vi "Write Clone name.vi"(8 "error in (no error)":errorcluster, 10 "Clone name":string, 11 "Fiber Auto Collimation panel in":refnum<class "Fiber Auto Collimation panel.lvclass">) -> (0 "error out":errorcluster, 3 "Fiber Auto Collimation panel out":refnum<class "Fiber Auto Collimation panel.lvclass">)   [LabVIEW 2018, in "Fiber Auto Collimation panel.lvclass"]
doc: "The \"Clone name\" is only needed if this is a Panel class that can be open more than once. If the panel will only be open once at a time, don't bother using this element of the private data for anything.\n\nClone names are forced into lower case and have whitespace removed from them when written. If the panel can be open more than once simultaneously, just be sure that each instance of the panel has a unique non-blank name.\n\nNote: The clone name should only be written during the panel launch and then propagated appropriately afterwards. Do not change the clone name after the panel has been started!"
uses:
  Fiber Auto Collimation panel.lvclass
  Fiber Auto Collimation panel.lvclass/Fiber Auto Collimation panel.ctl
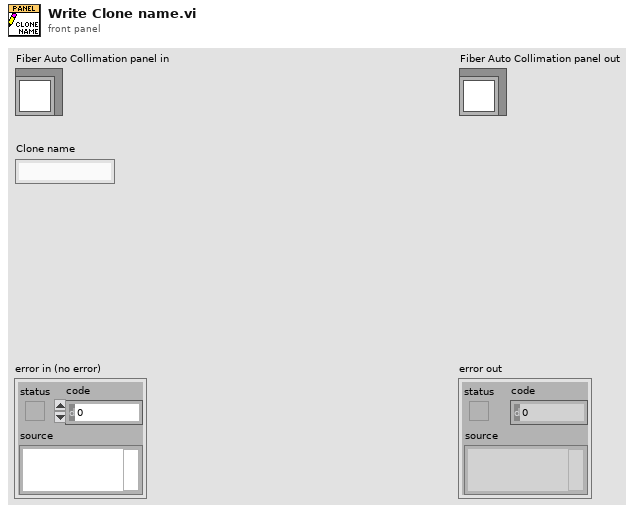
[diagram p1: front panel]
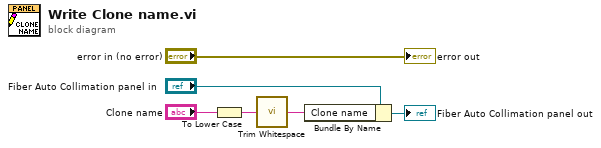
[diagram p0: block diagram]
diagram:
  n1 = To Lower Case(string="Clone name") -> (all lower case string=w2:string)
  n2 = call <vilib>:"Trim Whitespace.vi"("string"=w2) -> ("trimmed string"=w1:string)  [unwired: 1 in]
  n3 = Bundle By Name(cluster="Fiber Auto Collimation panel in", "Clone name"=w1) -> (→"Fiber Auto Collimation panel out":refnum<class "Fiber Auto Collimation panel.lvclass">)
  "error out" <- "error in (no error)"
